vi "Error Converter(ErrCheck).vi"(8 "error in (no error)":errorcluster, 10 "additional string":string="This error is returned by the shared library function.", 11 "status":i32) -> (0 "error out":errorcluster)   [LabVIEW 2026]
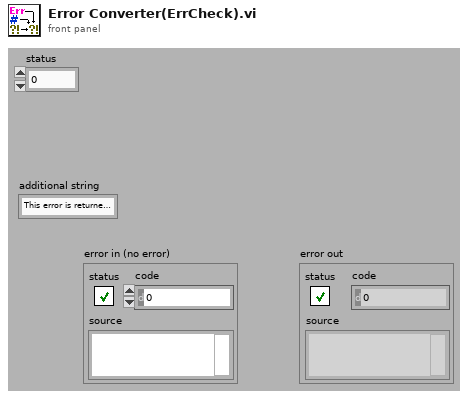
[diagram p1: front panel]
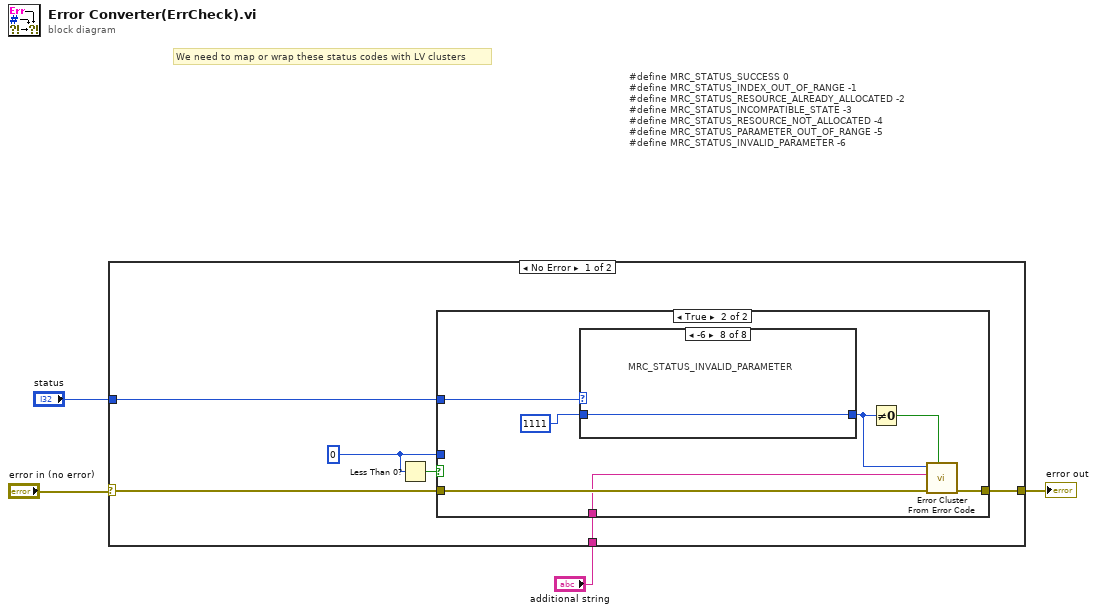
[diagram p0: block diagram]
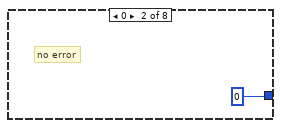
[diagram p4: hidden frame]
diagram:
  # "We need to map or wrap these status codes with LV clusters"
  # "#define MRC_STATUS_SUCCESS 0\n#define MRC_STATUS_INDEX_OUT_OF_RANGE -1\n#define MRC_STATUS_RESOURCE_ALREADY_ALLOCATED -2\n#define MRC_STATUS_INCOMPATIBLE_STATE -3\n#define MRC_STATUS_RESOURCE_NOT_ALLOCATED -4\n#define MRC_STATUS_PARAMETER_OUT_OF_RANGE -5\n#define MRC_STATUS_INVALID_PARAMETER -6"
  n1 = case shown="No Error" "error in (no error)" {
    selector: "error in (no error)" -> [w9 w27]
    tunnel: [w8 w27] -> w3
    tunnel: "status" -> [w6 _]
    tunnel: "additional string" -> [w5 _]
    frame No Error {
      w7 = 0 ("Error Code")
      n2 = Less Than 0?(x=w7) -> (x < 0?=w10:bool)
      n3 = case shown="True" w10 {
        tunnel: w9 -> [w11 w18]
        tunnel: w7 -> [_ _]
        tunnel: [w11 w17] -> w8
        tunnel: w6 -> [_ w16]
        tunnel: w5 -> [_ w15]
        frame False {
        }
        frame True {
          n4 = case shown="-6" w16 {
            tunnel: [w19 0 ("Error Code") w21 w22 w23 w24 w25 w26] -> w13
            tunnel: 1111 ("Error Code") -> [w19 _ w21 w22 w23 w24 w25 w26]
            frame Default {
              # "what is this"
            }
            frame 0 {
              # "no error"
            }
            frame -1 {
              # "MRC_STATUS_INDEX_OUT_OF_RANGE"
            }
            frame -2 {
              # "MRC_STATUS_RESOURCE_ALREADY_ALLOCATED"
            }
            frame -3 {
              # "MRC_STATUS_INCOMPATIBLE_STATE"
            }
            frame -4 {
              # "MRC_STATUS_RESOURCE_NOT_ALLOCATED"
            }
            frame -5 {
              # "MRC_STATUS_PARAMETER_OUT_OF_RANGE"
            }
            frame -6 {
              # "MRC_STATUS_INVALID_PARAMETER"
            }
          }
          n5 = Not Equal To 0?(x=w13) -> (x != 0?=w12:bool)
          n6 = call <vilib>:"Error Cluster From Error Code.vi"("show call chain? (False)"=w12, "error in (no error)"=w18, "error message (\"\")"=w15, "error code (0)"=w13) -> ("error out"=w17:errorcluster)  [unwired: 5 in]
        }
      }
    }
    frame Error {
    }
  }
  "error out" <- w3
